vi "UnitTestPractice.vi"(8 "error in (no error)":errorcluster, 9 "Numeric 2":dbl, 10 "Numeric":dbl, 11 "Operation":T1(ring)) -> (0 "error out":errorcluster, 2 "Result":dbl, 3 "String":string)   [LabVIEW 2018]
uses:
  <vilib>/Utility/error.llb/Error Cluster From Error Code.vi
  <vilib>/ErrorRing/Error Ring.xnode
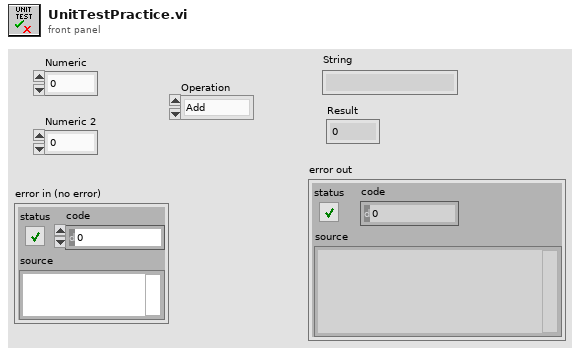
[diagram p1: front panel]
types:
  T1 = enum16{"Add", "Subtract", "Multiply", "Divide", "Inject Error"}
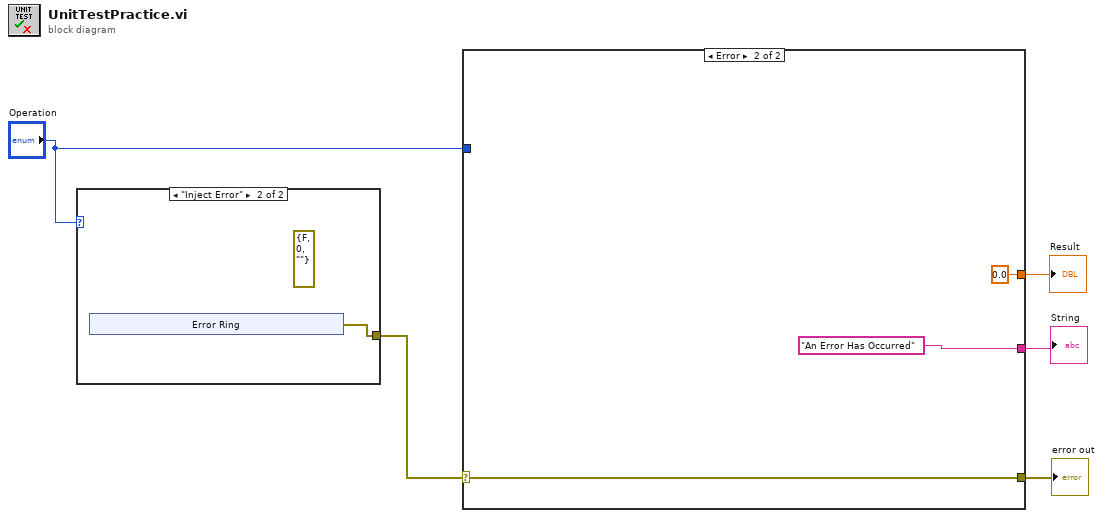
[diagram p0: block diagram]
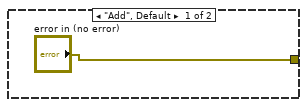
[diagram p2: hidden frame]
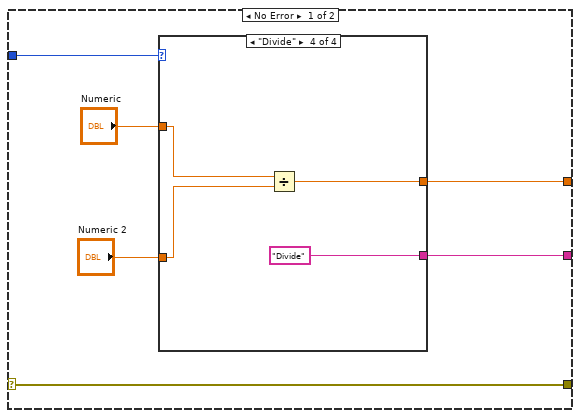
[diagram p3: hidden frame]
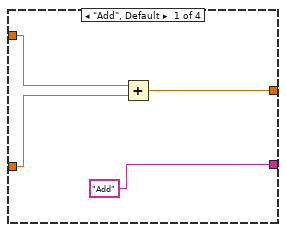
[diagram p4: hidden frame]
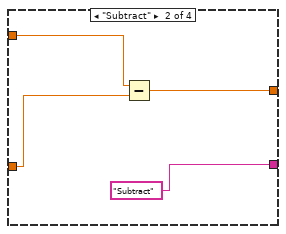
[diagram p5: hidden frame]
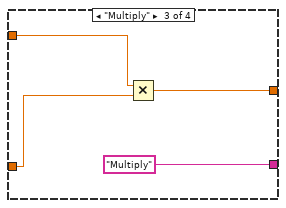
[diagram p6: hidden frame]
diagram:
  n1 = case shown="\"Inject Error\"" "Operation" {
    tunnel: ["error in (no error)" w7] -> w2
    frame "Add", Default {
    }
    frame "Inject Error" {
      (unwired) errorcluster {"status"=FALSE, "code"=0, "source"=""} ("error constant")
      n2 = xnode "Error Ring"() -> ("error out"=w7:errorcluster)
    }
  }
  n3 = case shown="Error" w2 {
    selector: w2 -> [w17 w36]
    tunnel: [w17 w36] -> w5
    tunnel: [w14 "An Error Has Occurred"] -> w4
    tunnel: [w13 0.0] -> w3
    tunnel: "Operation" -> [w12 _]
    frame No Error {
      n4 = case shown="\"Divide\"" w12 {
        tunnel: "Numeric" -> [w19 w23 w26 w32]
        tunnel: "Numeric 2" -> [w20 w24 w27 w33]
        tunnel: ["Add" "Subtract" "Multiply" "Divide"] -> w14
        tunnel: [w21 w22 w29 w30] -> w13
        frame "Add", Default {
          n5 = Add(x=w19, y=w20) -> (x+y=w21:dbl)
        }
        frame "Subtract" {
          n6 = Subtract(x=w23, y=w24) -> (x-y=w22:dbl)
        }
        frame "Multiply" {
          n7 = Multiply(x=w26, y=w27) -> (x*y=w29:dbl)
        }
        frame "Divide" {
          n8 = Divide(x=w32, y=w33) -> (x/y=w30:dbl)
        }
      }
    }
    frame Error {
    }
  }
  "error out" <- w5
  "String" <- w4
  "Result" <- w3
